vi "ReadTestItem.vi"(11 "GuiRef":T1={"StringOut"=refnum, "AbortOnFail"=refnum, "SN"=refnum, "SN_Length"=refnum, "TestResult"=refnum, "Starttime"=refnum, "CycleTime"=refnum, "ErrorCode"=refnum, "UUTStatus"=refnum, "DataBaseEnable?"=refnum, "DUTModel"=refnum, "FixtureID"=refnum, "OperatorID"=refnum, "SNReady"=refnum, "StopSlot"=refnum, "NextStep"=refnum, "SlotStart?"=refnum, "PassYeild"=refnum, "Failed"=refnum, "Passed"=refnum, "Tested"=refnum, "ErrorStop"=refnum, "SlotReady"=refnum, "StartTest"=refnum, "TestItemsCtl"={"StepName"="", "TestEnable"=FALSE, "LoopCount"=0, "StopOnFail"=FALSE, "LastStep?"=FALSE, "Index"=0, "TestName"="", "通道"="", "参数"="", "下限值"="", "上限值"="", "TimeStart"=0, "单位"=""}, "ProcessBar"=refnum, "Slot"=enum."Slot1", "Row"=3, "States"=refnum, "TestMode"=refnum, "PassYeild"=refnum, "ShowSkipStep?"=FALSE, "IniConfig"=refnum, "循环次数-DUT"=refnum, "DAQmx设备名"=refnum, "波形图"=refnum, "输入电压"=refnum, "产品型号"=refnum, "上电"=refnum, "测试项目"=refnum, "DAQConfigRef"=refnum, "子面板"=refnum, "测试结果"=refnum, "测试失败项目"=refnum, "开始按钮-DUT"=refnum, "Device ID"=0} {"Device ID" format="%.0x"}) -> ()   [LabVIEW 2013]
uses:
  <vilib>/Utility/file.llb/Read From Spreadsheet File (string).vi
  SysControl/Reference.ctl
  SysControl/TestItemsCTL.ctl
  SysControl/Slot.ctl
  Controls/DAQConfig.ctl
  Controls/DAQConfigRef.ctl
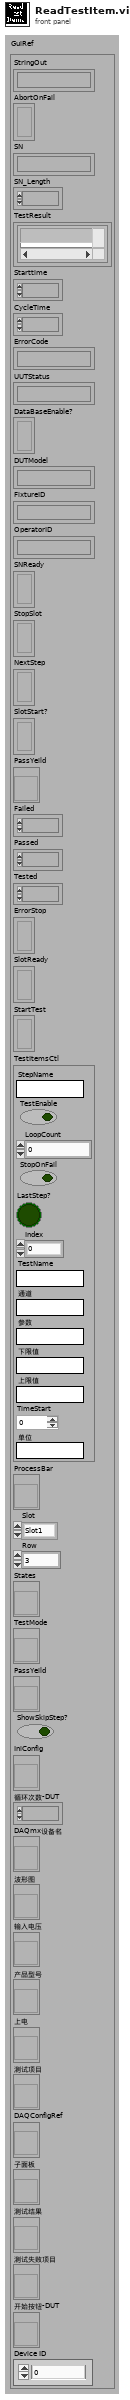
[diagram p1: front panel]
types:
  T1 = typedef "Reference.ctl" = cluster{"StringOut":refnum<vi>, "AbortOnFail":refnum<vi>, "SN":refnum<vi>, "SN_Length":refnum<vi>, "TestResult":refnum<vi>, "Starttime":refnum<vi>, "CycleTime":refnum<vi>, "ErrorCode":refnum<vi>, "UUTStatus":refnum<vi>, "DataBaseEnable?":refnum<vi>, "DUTModel":refnum<vi>, "FixtureID":refnum<vi>, "OperatorID":refnum<vi>, "SNReady":refnum<vi>, "StopSlot":refnum<vi>, "NextStep":refnum<vi>, "SlotStart?":refnum<vi>, "PassYeild":refnum<vi>, "Failed":refnum<vi>, "Passed":refnum<vi>, "Tested":refnum<vi>, "ErrorStop":refnum<vi>, "SlotReady":refnum<vi>, "StartTest":refnum<vi>, "TestItemsCtl":T2, "ProcessBar":refnum<vi>, "Slot":T3, "Row":i32, "States":refnum<vi>, "TestMode":refnum<vi>, "PassYeild":refnum<vi>, "ShowSkipStep?":bool, "IniConfig":refnum<vi>, "循环次数-DUT":refnum<vi>, "DAQmx设备名":refnum<vi>, "波形图":refnum<vi>, "输入电压":refnum<vi>, "产品型号":refnum<vi>, "上电":refnum<vi>, "测试项目":refnum<vi>, "DAQConfigRef":T4, "子面板":refnum<vi>, "测试结果":refnum<vi>, "测试失败项目":refnum<vi>, "开始按钮-DUT":refnum<vi>, "Device ID":u32}
  T2 = typedef "TestItemsCTL.ctl" = cluster{"StepName":string, "TestEnable":bool, "LoopCount":i32, "StopOnFail":bool, "LastStep?":bool, "Index":i32, "TestName":string, "通道":string, "参数":string, "下限值":string, "上限值":string, "TimeStart":u32, "单位":string}
  T3 = typedef "Slot.ctl" = enum16{"Slot1", "Slot2", "Slot3", "Slot4"}
  T4 = typedef "DAQConfigRef.ctl" = refnum<vi>
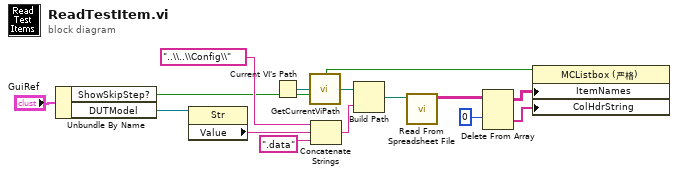
[diagram p0: block diagram]
diagram:
  n1 = Unbundle By Name("GuiRef") -> ("ShowSkipStep?"=w5:bool, "DUTModel"=w4:refnum<vi>)
  n2 = property class="Str"(reference=w4) -> ("Value"=w3:string)  [unwired: 1 in, 2 out]
  n3 = Current VI's Path() -> (path=w2:path)
  n4 = call "GetCurrentViPath.vi"("PathIn"=w2) -> ("CurrentViPath"=w1:path)
  n5 = Concatenate Strings("..\\..\\Config\\" ("字符串"), w3, ".data" ("字符串")) -> (w12:string)
  n6 = Build Path(base path=w1, name or relative path=w12) -> (appended path=w11:path)
  n7 = call-poly <vilib>:"Read From Spreadsheet File.vi"("file path (dialog if empty)"=w11) -> ("all rows"=w9:string[][])  [unwired: 3 in, 7 out]
  n8 = Delete From Array(array=w9, index (row)=0 ("索引 (行)")) -> (deleted portion=w8:string[], array with subset deleted=w7:string[][])  [unwired: 2 in]
  n9 = property on="属性节点" class="MCListbox (严格)"(reference=w5, "ItemNames"=w7, "ColHdrString"=w8) -> ()  [unwired: 1 in, 2 out]
